vi "case according to command.vi"(8 "error in":errorcluster, 11 "command":T1=22 items=["NO_Action", "start", "pause", "resum", "stop", "config", "System_constant", "7", "DAQ_init", "DAQ_config", "DAQ_start", "DAQ_read", "DAQ_stop", "DAQ_contrl", "14", "15", "16", "17", "18", "19", "Zsf_open", "Zsf_close", "Wkf_control", "Pump_switch", "dcf_switch", "JRQ_switch"]) -> (0 "error out":errorcluster, 2 "case":string="Command - Wkf_control")   [LabVIEW 2011]
uses:
  Ctrls/command.ctl
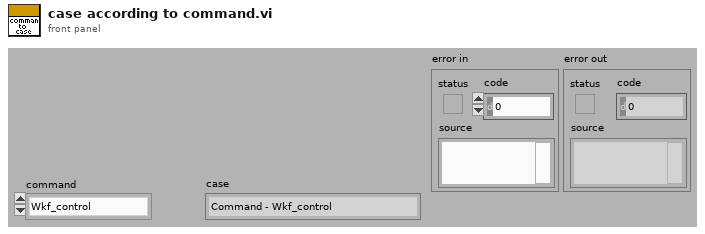
[diagram p1: front panel]
types:
  T1 = typedef "command.ctl" = u16
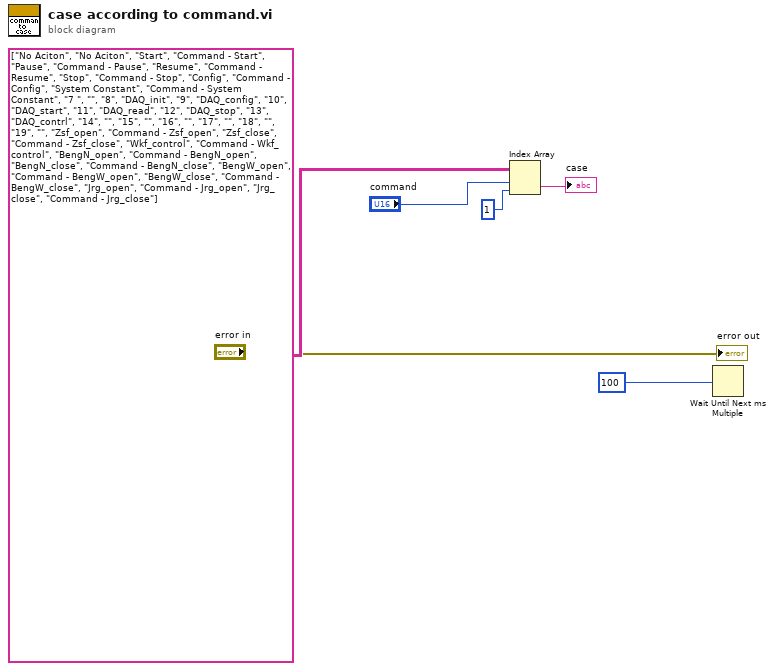
[diagram p0: block diagram]
diagram:
  n1 = Index Array(array=string[][] [["No Aciton", "No Aciton"], ["Start", "Command - Start"], ["Pause", "Command - Pause"], ["Resume", "Command - Resume"], ["Stop", "Command - Stop"], ["Config", "Command - Config"], ["System Constant", "Command - System Constant"], ["7 ", ""], ["8", "DAQ_init"], ["9", "DAQ_config"], ["10", "DAQ_start"], ["11", "DAQ_read"], ["12", "DAQ_stop"], ["13", "DAQ_contrl"], ["14", ""], ["15", ""], ["16", ""], ["17", ""], ["18", ""], ["19", ""], ["Zsf_open", "Command - Zsf_open"], ["Zsf_close", "Command - Zsf_close"], ["Wkf_control", "Command - Wkf_control"], ["BengN_open", "Command - BengN_open"], ["BengN_close", "Command - BengN_close"], ["BengW_open", "Command - BengW_open"], ["BengW_close", "Command - BengW_close"], ["Jrg_open", "Command - Jrg_open"], ["Jrg_close", "Command - Jrg_close"]] ("command to case"), index (row)="command", index (col)=1 ("disabled index (col)")) -> (element=→"case":string)
  n2 = Wait Until Next ms Multiple(millisecond multiple=u32 100) -> ()  [unwired: 1 out]
  "error out" <- "error in"
